vi "DrawOnStage.vi"(3 "error in":errorcluster, 4 "object in":refnum<vi>, 5 "Stage in":refnum<vi>) -> (0 "error out":errorcluster, 1 "Object out":refnum<vi>, 2 "Stage out":refnum<vi>)   [LabVIEW 2024]
uses:
  <vilib>/picture/3D Picture Control/Object/Create Object (name).vi
  <vilib>/picture/3D Picture Control/NI_3D Picture Control.lvlib
panel:
  in  "Name":string="Undec"
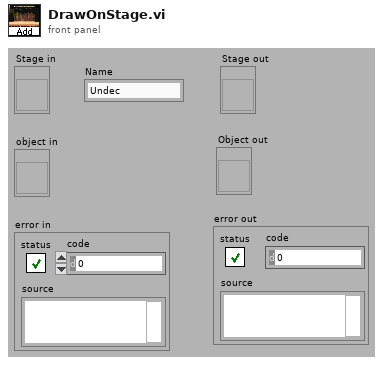
[diagram p1: front panel]
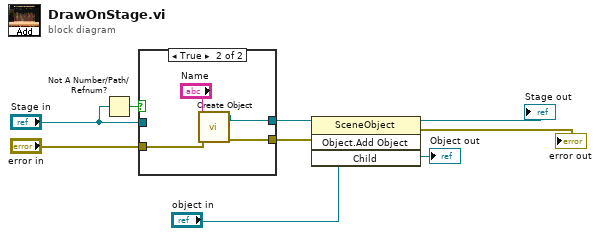
[diagram p0: block diagram]
diagram:
  n1 = Not A Number/Path/Refnum?(number/path/refnum="Stage in") -> (NaN/Path/Refnum?=w6:bool)
  n2 = case shown="True" w6 {
    tunnel: "error in" -> [w10 w14]
    tunnel: [w10 w13] -> w4
    tunnel: [w11 w12] -> w3
    tunnel: "Stage in" -> [w11 _]
    frame False {
    }
    frame True {
      n3 = call-poly <vilib>:"Create Object.vi"("error in (no error)"=w14, "Name"="Name") -> ("error out"=w13:errorcluster, "Scene:New Object"=w12:refnum<vi>)  [unwired: 8 in]
    }
  }
  n4 = invoke class="SceneObject" method="Object.Add Object"(reference=w3, error in=w4, "Child"="object in") -> (reference out=→"Stage out":refnum<vi>, error out=→"error out":errorcluster, "Child"=→"Object out":refnum<vi>)  [unwired: 1 in, 1 out]
